vi "CalcWavelength.vi"(1 "Grating":enum16{"1200", "600", "300"}(ring), 2 "Grating Wavelength (nm)":dbl format="%#_6p") -> (0 "Wavelength array":dbl[](array[numeric]) format="%_15p")   [LabVIEW 2009]
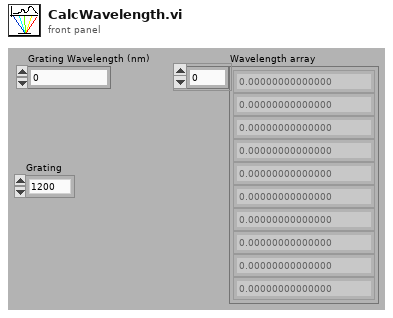
[diagram p1: front panel]
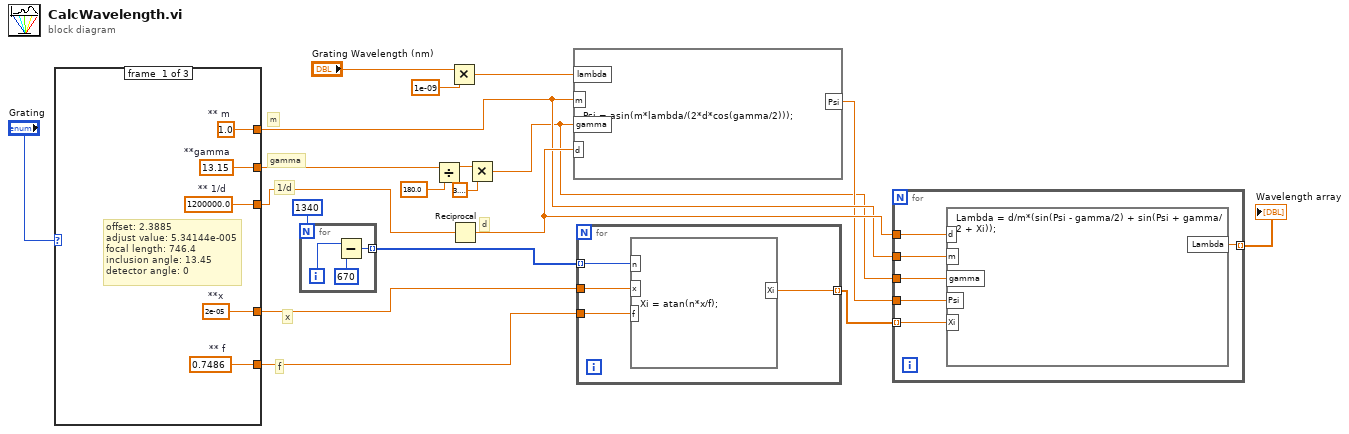
[diagram p0: block diagram]
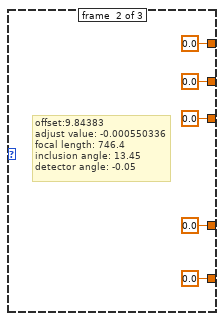
[diagram p2: hidden frame]
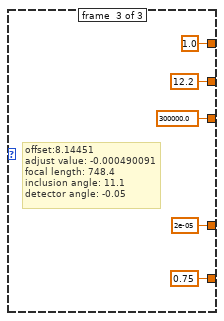
[diagram p3: hidden frame]
diagram:
  # "f"
  # "x"
  # "1/d"
  # "gamma"
  # "m"
  # "d"
  n1 = case shown="\"300\"" "Grating" {
    tunnel: [w24 0.0 ("**gamma") 12.2 ("**gamma")] -> w19
    tunnel: [w23 0.0 ("** f") 0.75 ("** f")] -> w13
    tunnel: [w22 0.0 ("**x") 2e-05 ("**x")] -> w12
    tunnel: [w21 0.0 ("** m") 1.0 ("** m")] -> w8
    tunnel: [w20 0.0 ("** 1/d") 300000.0 ("** 1/d")] -> w2
    frame #0 {
      w22 = 2e-05  # **x
      w23 = 0.7486  # ** f
      w24 = 13.15  # **gamma
      w21 = 1.0  # ** m
      w20 = 1200000.0  # ** 1/d
      # "offset: 2.3885\nadjust value: 5.34144e-005\nfocal length: 746.4\ninclusion angle: 13.45\ndetector angle: 0"
    }
    frame #1 {
      # "offset:9.84383\nadjust value: -0.000550336\nfocal length: 746.4\ninclusion angle: 13.45\ndetector angle: -0.05"
    }
    frame #2 {
      # "offset:8.14451\nadjust value: -0.000490091\nfocal length: 748.4\ninclusion angle: 11.1\ndetector angle: -0.05"
    }
  }
  n2 = for {
    N: 1340 -> [_]
    tunnel: [w35] -> w11 mode=indexing
    i -> [w37]
    n3 = Subtract(x=w37, y=670) -> (x-y=w35:i32)
  }
  n4 = Divide(x=w19, y=180.0 ("** Gamma")) -> (x/y=w17:dbl)
  n5 = Multiply(x="Grating Wavelength (nm)", y=1e-09) -> (x*y=w5:dbl)
  n6 = Reciprocal(x=w2) -> (1/x=w9:dbl)
  n7 = Multiply(x=w17, y=3.141592653589793) -> (x*y=w6:dbl)
  n8 = formula code="Psi = asin(m*lambda/(2*d*cos(gamma/2)));"("lambda"=w5, "m"=w8, "d"=w9, "gamma"=w6) -> ("Psi"=w7:dbl)
  n9 = for {
    tunnel: w13 -> [w41]
    tunnel: w12 -> [w40]
    tunnel: w11 -> [w39] mode=indexing
    tunnel: [w38] -> w10 mode=indexing
    n10 = formula code="Xi = atan(n*x/f);"("n"=w39, "x"=w40, "f"=w41) -> ("Xi"=w38:dbl)
  }
  n11 = for {
    tunnel: w10 -> [w47] mode=indexing
    tunnel: w9 -> [w46]
    tunnel: w8 -> [w45]
    tunnel: w7 -> [w44]
    tunnel: w6 -> [w43]
    tunnel: [w42] -> w3 mode=indexing
    n12 = formula code="Lambda = d/m*(sin(Psi - gamma/2) + sin(Psi + gamma/2 + Xi));"("Xi"=w47, "d"=w46, "m"=w45, "Psi"=w44, "gamma"=w43) -> ("Lambda"=w42:dbl)
  }
  "Wavelength array" <- w3
